vi "TH_Print_Panel.vi"   [LabVIEW 2014]
uses:
  <vilib>/Utility/NIReport.llb/HTML Report Image Alignment.ctl
  <vilib>/Utility/NIReport.llb/NI_report.lvclass
  <vilib>/Utility/NIReport.llb/NI_ReportGenerationCore.lvlib
types:
  T1 = cluster{"top":dbl, "left":dbl, "right":dbl, "bottom":dbl}
  T2 = typedef "NI_ReportGenerationCore.lvlib/HTML Report Image Alignment.ctl" = enum16{"(default)", "LEFT", "RIGHT", "TOP", "TEXTTOP", "MIDDLE", "ABSMIDDLE", "BASELINE", "BOTTOM", "ABSBOTTOM"}
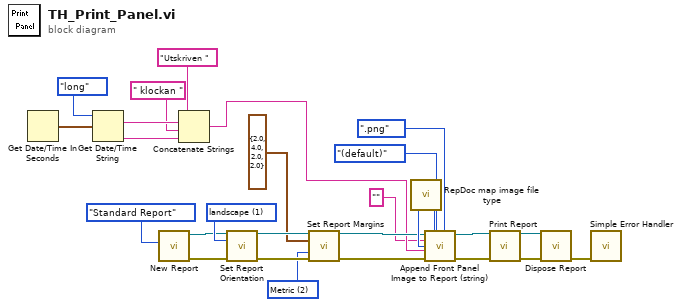
[diagram p0: block diagram]
diagram:
  w14 = u16 2 items=["Default", "US", "Metric"] ("measurement system (Default)")
  w21 = u16 1 items=["portrait", "landscape"] ("orientation (portrait)")
  n1 = Get Date/Time In Seconds() -> (seconds since 1Jan1904=w10:timestamp)
  n2 = Get Date/Time String(date format (0)=enum16{"short", "long", "abbreviated"}."long", seconds (now)=w10) -> (date string=w7:string, time string=w5:string)  [unwired: 1 in]
  n3 = call <vilib>:"New Report.vi"("report type"=enum16{"Standard Report", "HTML"}."Standard Report") -> ("report out"=w18:refnum<class "NI_report.lvclass">, "error out"=w19:errorcluster)  [unwired: 13 in]
  n4 = Concatenate Strings("Utskriven " ("description"), w7, " klockan " ("string"), w5) -> (w6:string)
  n5 = call-dynamic "Set Report Orientation.vi"("report in"=w18, "orientation (portrait)"=w21, "error in (no error)"=w19) -> ("report out"=w15:refnum<class "NI_report.lvclass">, "error out"=w16:errorcluster)  [unwired: 11 in]
  n6 = call-dynamic "Set Report Margins.vi"("report in"=w15, "margins (1.00)"=T1 {"top"=2.0, "left"=4.0, "right"=2.0, "bottom"=2.0}, "measurement system (default)"=w14, "error in (no error)"=w16) -> ("report out"=w12:refnum<class "NI_report.lvclass">, "error out"=w11:errorcluster)  [unwired: 9 in, 1 out]
  n7 = call <vilib>:"RepDoc map image file type.vi"("image file type (.jpg)"=enum16{".jpg", ".png"}.".png" ("image file type(.jpg)")) -> ("image format (jpeg)"=w2:enum32{"PNG", "JPEG", "GIF"})
  n8 = call <vilib>:"Append Front Panel Image to Report (string).vi"("report in"=w12, "alignment (default)"=HTML_Report_Image_Alignment."(default)", "image format (jpeg)"=w2, "VI"="", "description"=w6, "error in (no error)"=w11) -> ("report out"=w17:refnum<class "NI_report.lvclass">, "error out"=w3:errorcluster)  [unwired: 5 in, 3 out]
  n9 = call-dynamic "Print Report.vi"("report in"=w17, "error in (no error)"=w3) -> ("report out"=w22:refnum<class "NI_report.lvclass">, "error out"=w26:errorcluster)  [unwired: 12 in]
  n10 = call-dynamic "Dispose Report.vi"("report in"=w22, "error in (no error)"=w26) -> ("error out"=w23:errorcluster)  [unwired: 13 in]
  n11 = call <vilib>:"Simple Error Handler.vi"("error in (no error)"=w23) -> ()  [unwired: 4 in, 5 out]
